vi "求取MFCC及DMFCC.vi"(2 "s2":dbl, 3 "s1":dbl, 4 "xx":dbl[][](array[numeric])) -> (0 "cof":dbl[][](array[numeric]), 1 "ccc":dbl[][](array[numeric]))   [LabVIEW 2018]
panel:
  out "error out":errorcluster
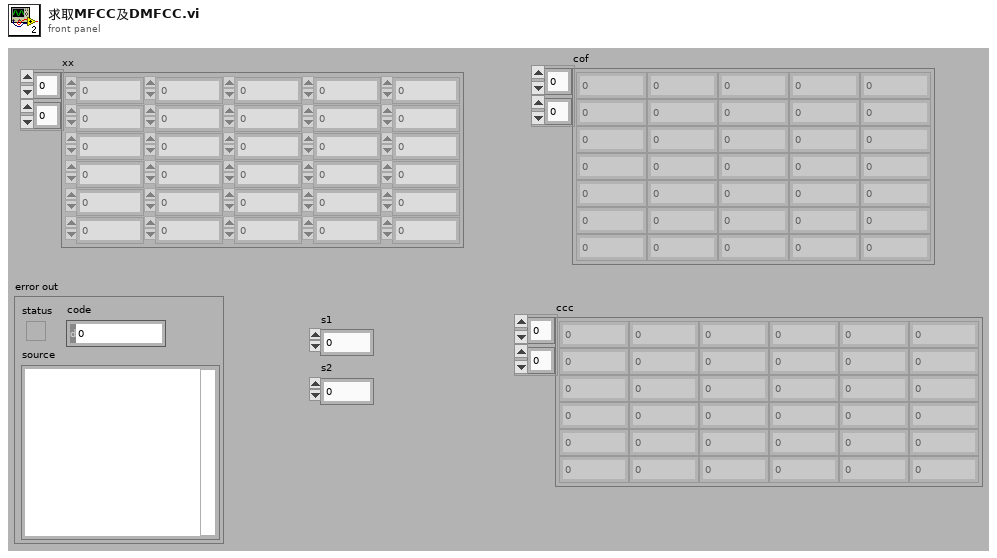
[diagram p1: front panel]
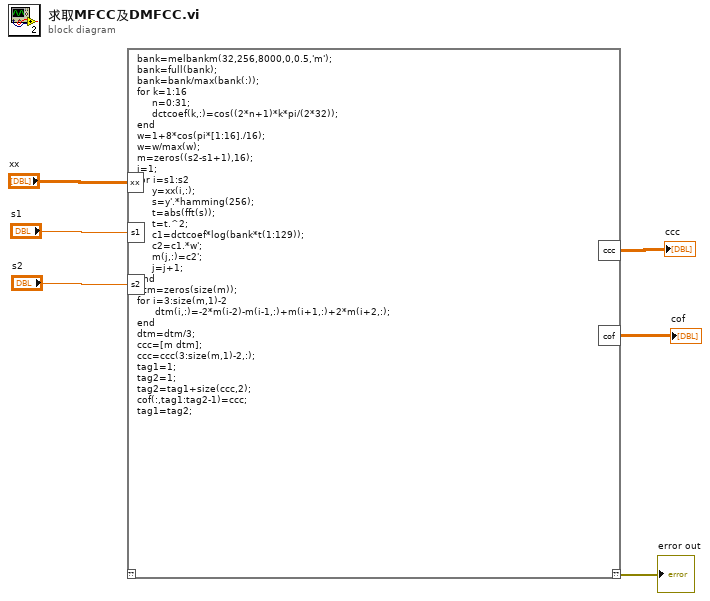
[diagram p0: block diagram]
diagram:
  n1 = script code="bank=melbankm(32,256,8000,0,0.5,'m');\nbank=full(bank);\nbank=bank/max(bank(:));\nfor k=1:16\n     n=0:31;\n     dctcoef(k,:)=cos((2*n+1)*k*pi/(2*32));\nend\nw=1+8*cos(pi*[1:16]./16);\nw=w/max(w);\nm=zeros((s2-s1+1),16);\nj=1;\nfor i=s1:s2\n     y=xx(i,:);\n     s=y'.*hamming(256);\n     t=abs(fft(s));\n     t=t.^2;\n     c1=dctcoef*log(bank*t(1:129));\n     c2=c1.*w';\n     m(j,:)=c2';\n     j=j+1;\nend\ndtm=zeros(size(m));\nfor i=3:size(m,1)-2\n      dtm(i,:)=-2*m(i-2)-m(i-1,:)+m(i+1,:)+2*m(i+2,:);\nend\ndtm=dtm/3;\nccc=[m dtm];\nccc=ccc(3:size(m,1)-2,:);\ntag1=1;\ntag2=1; \ntag2=tag1+size(ccc,2);\ncof(:,tag1:tag2-1)=ccc;\ntag1=tag2;"("xx"="xx", "s1"="s1", "s2"="s2") -> ("??"=→"error out":errorcluster, "ccc"=→"ccc":dbl[][], "cof"=→"cof":dbl[][])  [unwired: 1 in]
